vi "TargetAngle.vi"(10 "Tx in":dbl, 11 "Dist. From Target[in.] in":dbl) -> (1 "Angle of Target":dbl, 2 "hypoteneuse":dbl, 3 "Dist. From Target[in.] out":dbl, 4 "tx out":dbl)   [LabVIEW 2019]
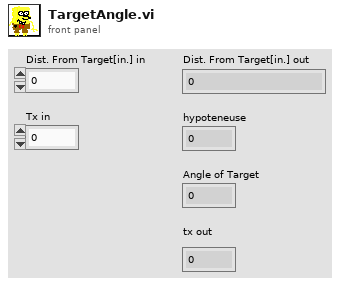
[diagram p1: front panel]
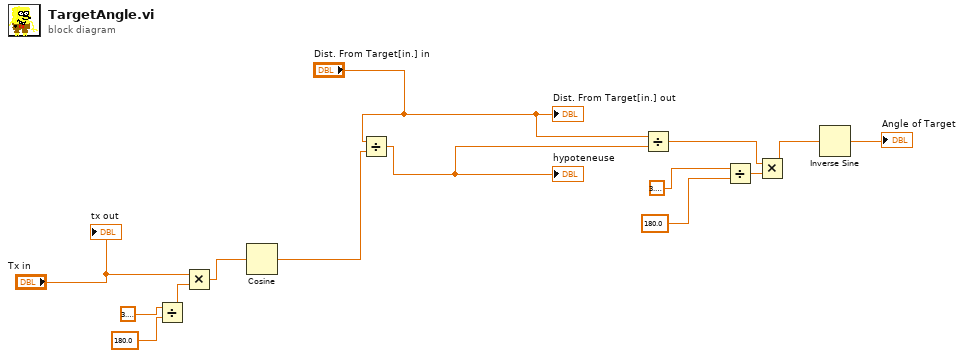
[diagram p0: block diagram]
diagram:
  n1 = Divide(x=3.141592653589793, y=180.0) -> (x/y=w3:dbl)
  n2 = Multiply(x="Tx in", y=w3) -> (x*y=w9:dbl)
  n3 = Cosine(x=w9) -> (cos(x)=w11:dbl)
  n4 = Divide(x="Dist. From Target[in.] in", y=w11) -> (x/y=w13:dbl)
  "hypoteneuse" <- w13
  n5 = Divide(x="Dist. From Target[in.] in", y=w13) -> (x/y=w7:dbl)
  n6 = Divide(x=3.141592653589793, y=180.0) -> (x/y=w4:dbl)
  n7 = Multiply(x=w7, y=w4) -> (x*y=w8:dbl)
  n8 = Inverse Sine(1:w8) -> (0:→"Angle of Target":dbl)
  "Dist. From Target[in.] out" <- "Dist. From Target[in.] in"
  "tx out" <- "Tx in"
